vi "Create All Message Queues.vi"(8 "error in":errorcluster) -> (0 "error out":errorcluster, 3 "Queues":T1)   [LabVIEW 2015, in "Message Queue.lvlib"]
doc: "Creates and initializes message queues"
uses:
  Message Queue.lvlib
  All Message Queues.ctl
  Message Cluster.ctl
  Enqueue Message (Single).vi
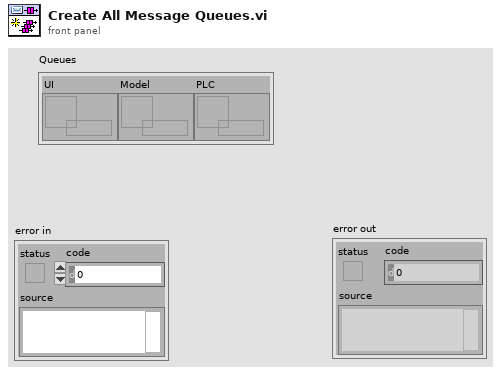
[diagram p1: front panel]
types:
  T1 = typedef "Message Queue.lvlib/All Message Queues.ctl" = cluster{"UI":refnum<queue>, "Model":refnum<queue>, "PLC":refnum<queue>}
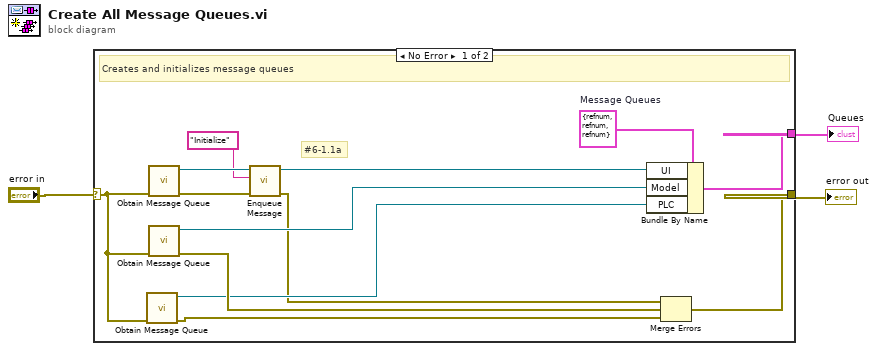
[diagram p0: block diagram]
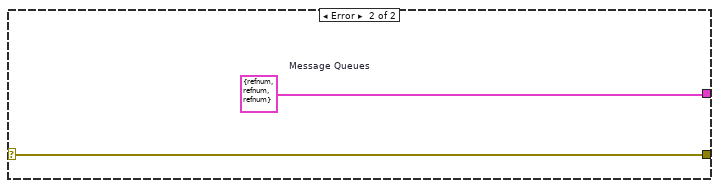
[diagram p2: hidden frame]
diagram:
  n1 = case shown="No Error" "error in" {
    selector: "error in" -> [w13 w18]
    tunnel: [w14 w18] -> w3
    tunnel: [w15 w17] -> w2
    frame No Error {
      w16 = T1 {"UI"=refnum, "Model"=refnum, "PLC"=refnum}  # Message Queues
      # "#6-1.1a"
      # "Creates and initializes message queues"
      n2 = call "Obtain Message Queue.vi"("error in (no error)"=w13) -> ("error out"=w10:errorcluster, "Message Queue"=w9:refnum<queue>)  [unwired: 9 in]
      n3 = call "Obtain Message Queue.vi"("error in (no error)"=w13) -> ("error out"=w7:errorcluster, "Message Queue"=w8:refnum<queue>)  [unwired: 9 in]
      n4 = call "Obtain Message Queue.vi"("error in (no error)"=w13) -> ("error out"=w12:errorcluster, "Message Queue"=w11:refnum<queue>)  [unwired: 9 in]
      n5 = call-poly "Enqueue Message.vi"("error in (no error)"=w7, "Message"="Initialize", "Message Queue"=w8) -> ("error out"=w6:errorcluster, "dup Message Queue"=w5:refnum<queue>)  [unwired: 7 in]
      n6 = Bundle By Name(cluster=w16, "UI"=w5, "Model"=w11, "PLC"=w9) -> (w15:T1)
      n7 = Merge Errors(w6, w12, w10) -> (w14:errorcluster)
    }
    frame Error {
      w17 = T1 {"UI"=refnum, "Model"=refnum, "PLC"=refnum}  # Message Queues
    }
  }
  "Queues" <- w2
  "error out" <- w3
